vi "Explorer_ReadConsole.vi"(6 "Reading":enum16{"Next", "Last"}(ring), 8 "index in":i32, 11 "String in":refnum<vi>) -> (0 "index out":i32, 1 "New Line":string, 2 "New point?":bool, 3 "String out":refnum<vi>, 5 "Value":string)   [LabVIEW 2022 SP3]
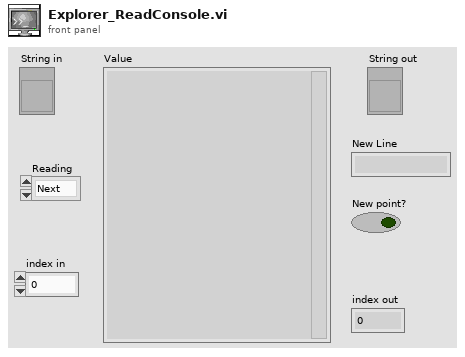
[diagram p1: front panel]
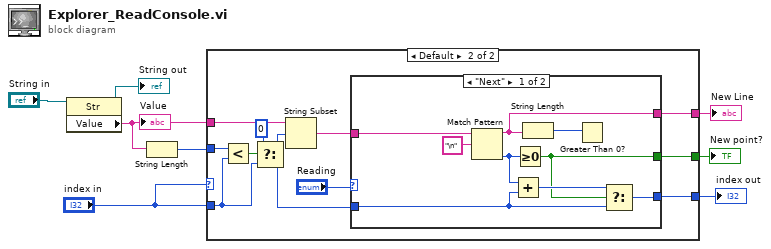
[diagram p0: block diagram]
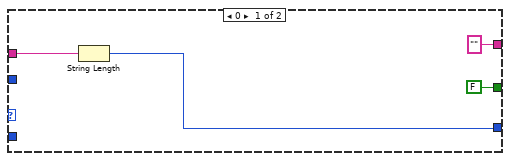
[diagram p2: hidden frame]
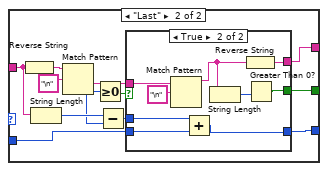
[diagram p3: hidden frame]
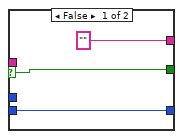
[diagram p4: hidden frame]
diagram:
  n1 = property class="Str"(reference="String in") -> (reference out=→"String out":refnum<vi>, "Value"=w2:string)  [unwired: 1 in, 1 out]
  "Value" <- w2
  n2 = String Length(string=w2) -> (length=w1:i32)
  n3 = case shown="Default" "index in" {
    tunnel: [FALSE w23] -> w8
    tunnel: "index in" -> [_ w15]
    tunnel: [w9 w22] -> w7
    tunnel: w2 -> [w10 w20]
    tunnel: ["" ("Value") w19] -> w5
    tunnel: w1 -> [_ w18]
    frame 0 {
      n4 = String Length(string=w10) -> (length=w9:i32)
    }
    frame Default {
      n5 = Less?(x=w18, y=w15) -> (x < y?=w17:bool)
      n6 = Select(t=0, s=w17, f=w15) -> (s? t:f=w14:i32)
      n7 = String Subset(string=w20, offset (0)=w14) -> (substring=w21:string)  [unwired: 1 in]
      n8 = case shown="\"Next\"" "Reading" {
        tunnel: [w24 w39] -> w23
        tunnel: [w30 w41] -> w22
        tunnel: w21 -> [w28 w36]
        tunnel: [w26 w38] -> w19
        tunnel: w14 -> [w27 w40]
        frame "Next" {
          n9 = Match Pattern(string=w28, regular expression="\n") -> (before substring=w26:string, offset past match=w31:i32)  [unwired: 1 in, 2 out]
          n10 = Add(x=w31, y=w27) -> (x+y=w32:i32)
          n11 = Greater Or Equal To 0?(x=w31) -> (x >= 0?=w24:bool)
          n12 = String Length(string=w26) -> (length=w25:i32)
          n13 = Greater Than 0?(x=w25) -> ()  [unwired: 1 out]
          n14 = Select(t=w32, s=w24, f=w27) -> (s? t:f=w30:i32)
        }
        frame "Last" {
          n15 = Reverse String(1:w36) -> (0:w43:string)
          n16 = String Length(string=w36) -> (length=w35:i32)
          n17 = Match Pattern(string=w43, regular expression="\n") -> (after substring=w37:string, offset past match=w34:i32)  [unwired: 1 in, 2 out]
          n18 = Greater Or Equal To 0?(x=w34) -> (x >= 0?=w42:bool)
          n19 = Subtract(x=w35, y=w34) -> (x-y=w33:i32)
          n20 = case shown="True" w42 {
            selector: w42 -> [w46 _]
            tunnel: [w47 w53] -> w41
            tunnel: w40 -> [w47 w54]
            tunnel: [w46 w48] -> w39
            tunnel: ["" ("regular expression") w51] -> w38
            tunnel: w37 -> [_ w56]
            tunnel: w33 -> [_ w55]
            frame False {
            }
            frame True {
              n21 = Match Pattern(string=w56, regular expression="\n") -> (before substring=w50:string)  [unwired: 1 in, 3 out]
              n22 = Add(x=w55, y=w54) -> (x+y=w53:i32)
              n23 = String Length(string=w50) -> (length=w49:i32)
              n24 = Reverse String(1:w50) -> (0:w51:string)
              n25 = Greater Than 0?(x=w49) -> (x > 0?=w48:bool)
            }
          }
        }
      }
    }
  }
  "New point?" <- w8
  "index out" <- w7
  "New Line" <- w5
